vi "Global 1.vi"() -> ()   [LabVIEW 2010]
panel:
  in  "Current State":string
  in  "Green Start Time (ms)":u32
  in  "Global Stop":bool
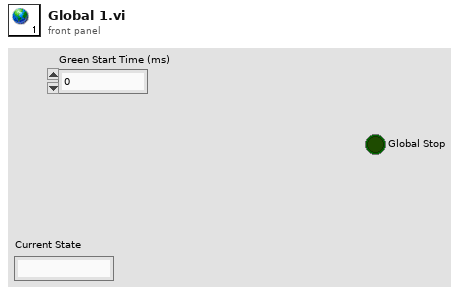
[diagram p1: front panel]
diagram:
